vi "byte_array_to_fixpoint_FPGA.vi"(11 "Array":u8[](array[numeric])=[0, 0, 0, 0]) -> (3 "y":fxp<+/-,32,9>)   [LabVIEW 2016]
uses:
  <vilib>/rvi/FXPMathLib/FxpConvert/subVIs/nifxpmath_Convert_SimConfig.ctl
  <vilib>/fxp/LVFixedPointQuantizationPolicyTypeDef.ctl
  <vilib>/fxp/LVFixedPointOverflowPolicyTypeDef.ctl
  <vilib>/rvi/FXPMathLib/FxpConvert/simVIs/DllFxpConvertTemp_sub.vi
  <vilib>/rvi/FXPMathLib/FxpConvert/XNode/nifxpmath_Convert.xnode
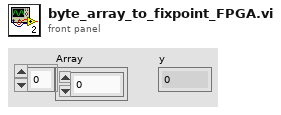
[diagram p1: front panel]
types:
  T1 = cluster{"Array[0]":u8, "Array[1]":u8, "Array[2]":u8, "Array[3]":u8}
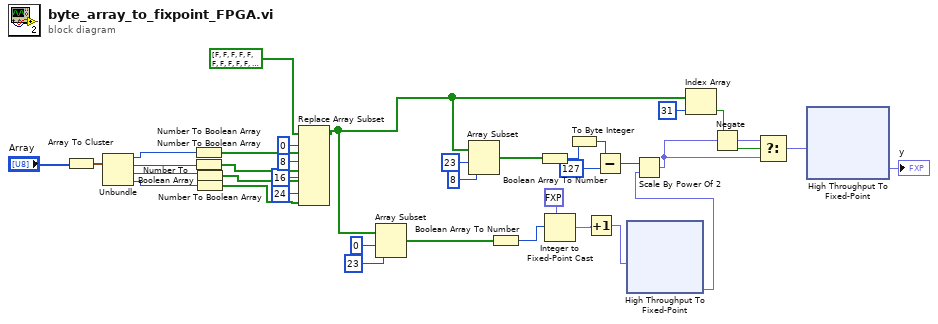
[diagram p0: block diagram]
diagram:
  n1 = Array To Cluster(array="Array") -> (cluster=w23:T1)
  n2 = Unbundle(w23) -> ("Array[0]"=w11:u8, "Array[1]"=w10:u8, "Array[2]"=w9:u8, "Array[3]"=w8:u8)
  n3 = Number To Boolean Array(number=w11) -> (Boolean array=w18:bool[])
  n4 = Number To Boolean Array(number=w10) -> (Boolean array=w17:bool[])
  n5 = Number To Boolean Array(number=w9) -> (Boolean array=w16:bool[])
  n6 = Number To Boolean Array(number=w8) -> (Boolean array=w15:bool[])
  n7 = Replace Array Subset(array=bool[] [FALSE, FALSE, FALSE, FALSE, FALSE, FALSE, FALSE, FALSE, FALSE, FALSE, FALSE, FALSE, FALSE, FALSE, FALSE, FALSE, FALSE, FALSE, FALSE, FALSE, FALSE, FALSE, FALSE, FALSE, FALSE, FALSE, FALSE, FALSE, FALSE, FALSE, FALSE, FALSE], new element #1=w18, index #1=0 ("index"), new element #2=w17, index #2=8 ("index"), new element #3=w16, index #3=16 ("index"), new element #4=w15, index #4=24 ("index")) -> (w13:bool[])
  n8 = Array Subset(array=w13, index=0, length=23) -> (w7:bool[])
  n9 = Array Subset(array=w13, index=23, length=8) -> (w1:bool[])
  n10 = Boolean Array To Number(Boolean array=w7) -> (number=w35:u32)
  n11 = Boolean Array To Number(Boolean array=w1) -> (number=w4:u8)
  n12 = Integer to Fixed-Point Cast(fixed-point type=fxp<+,23,0> 0.0, integer=w35) -> (fixed-point=w32:fxp<+,23,0>)
  n13 = To Byte Integer(number=w4) -> (8bit integer=w3:i8)
  n14 = Increment(x=w32) -> (x+1=w34:fxp<+,24,1>)
  n15 = Subtract(x=w3, y=i8 127) -> (x-y=w5:i8)
  n16 = xnode "High Throughput To Fixed-Point"("x"=w34) -> ("y"=w6:fxp<+/-,32,9>)
  n17 = Scale By Power Of 2(n=w5, x=w6) -> (x*2^n=w33:fxp<+/-,32,9>)
  n18 = Index Array(array=w13, index=31) -> (element=w25:bool)
  n19 = Negate(x=w33) -> (-x=w26:fxp<+/-,33,10>)
  n20 = Select(t=w26, s=w25, f=w33) -> (s? t:f=w36:fxp<+/-,33,10>)
  n21 = xnode "High Throughput To Fixed-Point"("x"=w36) -> ("y"=→"y":fxp<+/-,32,9>)
